vi "Sort Array.vi"(1 "Array In":dbl[](array[numeric])) -> (0 "Sorted Array Out":dbl[](array[numeric]))   [LabVIEW 2015]
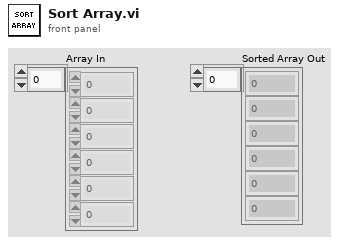
[diagram p1: front panel]
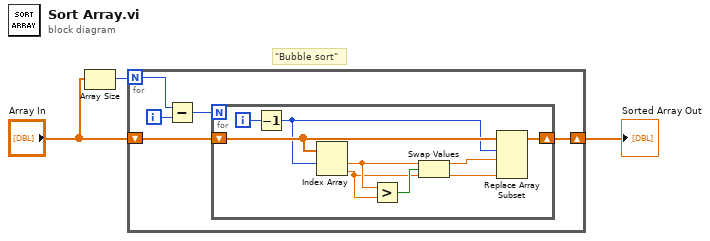
[diagram p0: block diagram]
diagram:
  # "\"Bubble sort\""
  n1 = Array Size(array="Array In") -> (size(s)=w1:i32)
  n2 = for {
    N: w1 -> [w7]
    shift-right: [w8] -> w3
    shift-left: "Array In" -> [w4]
    i -> [w5]
    n3 = Subtract(x=w7, y=w5) -> (x-y=w6:i32)
    n4 = for {
      N: w6 -> [_]
      shift-right: [w12] -> w8
      shift-left: w4 -> [w13]
      i -> [w17]
      n5 = Decrement(x=w17) -> (x-1=w11:i32)
      n6 = Index Array(array=w13, index #1=w11) -> (element #1=w15:dbl, element #2=w14:dbl)  [unwired: 1 in]
      n7 = Greater?(x=w15, y=w14) -> (0:w16:bool)
      n8 = Swap Values(12:w15, 13:w16, 14:w14) -> (1:w10:dbl, 3:w9:dbl)
      n9 = Replace Array Subset(array=w13, new element #1=w10, index #1=w11, new element #2=w9) -> (w12:dbl[])  [unwired: 1 in]
    }
  }
  "Sorted Array Out" <- w3
